vi "Get Channels From Configuration.vi"(8 "error in (no error)":errorcluster, 11 "Path":path=path "C:/Gas Circulation Tester/Configuration/Channels.txt") -> (0 "error out":errorcluster, 3 "Channels":T1[](array[typedef]))   [LabVIEW 2015]
doc: "This VI gets a channel list from a configuration file. The Input string must be comma delimited"
uses:
  Controls/Channel Configuration.ctl
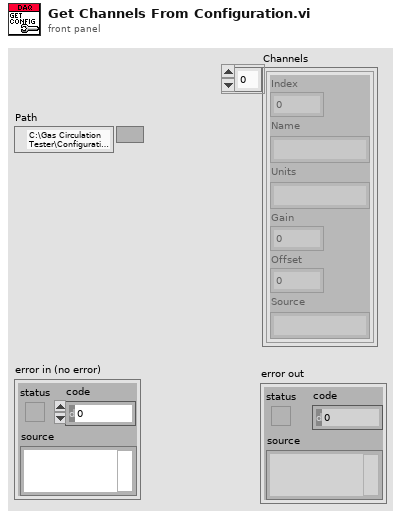
[diagram p1: front panel]
types:
  T1 = typedef "Channel Configuration.ctl" = cluster{"Index":u16, "Name":string, "Units":string, "Gain":dbl, "Offset":dbl, "Source":string}
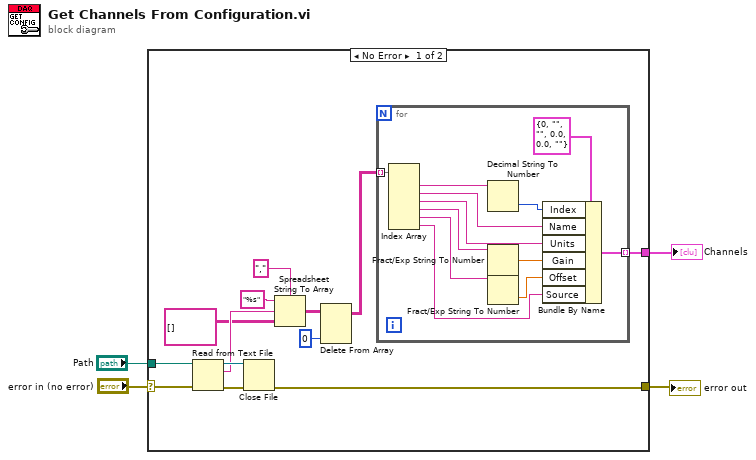
[diagram p0: block diagram]
diagram:
  n1 = case shown="No Error" "error in (no error)" {
    selector: "error in (no error)" -> [w17 w30]
    tunnel: [w9 w30] -> w4
    tunnel: "Path" -> [w16 _]
    tunnel: [w5 _] -> w1
    frame No Error {
      n2 = Read from Text File(file (use dialog)=w16, error in=w17) -> (refnum out=w14:refnum<file>, text=w13:string, error out=w15:errorcluster)  [unwired: 2 in, 1 out]
      n3 = Close File(refnum=w14, error in=w15) -> (error out=w9:errorcluster)  [unwired: 1 out]
      n4 = Spreadsheet String To Array(delimiter (Tab)=",", format string="%s", spreadsheet string=w13, array type (2D Dbl)=string[][] []) -> (array=w8:string[][])
      n5 = Delete From Array(array=w8, index (row)=0) -> (array with subset deleted=w6:string[][])  [unwired: 2 in, 1 out]
      n6 = for {
        tunnel: w6 -> [w29] mode=indexing
        tunnel: [w18] -> w5 mode=indexing
        n7 = Index Array(array=w29) -> (element #1=w27:string, element #2=w25:string, element #3=w24:string, element #4=w22:string, element #5=w21:string, element #6=w19:string)  [unwired: 6 in]
        n8 = Decimal String To Number(string=w27) -> (number=w26:i32)  [unwired: 2 in, 1 out]
        n9 = Fract/Exp String To Number(string=w22) -> (number=w23:dbl)  [unwired: 3 in, 1 out]
        n10 = Fract/Exp String To Number(string=w21) -> (number=w20:dbl)  [unwired: 3 in, 1 out]
        n11 = Bundle By Name(cluster=T1 {"Index"=0, "Name"="", "Units"="", "Gain"=0.0, "Offset"=0.0, "Source"=""} ("Channel Config"), "Index"=w26, "Name"=w25, "Units"=w24, "Gain"=w23, "Offset"=w20, "Source"=w19) -> (w18:T1)
      }
    }
    frame Error {
    }
  }
  "error out" <- w4
  "Channels" <- w1
